vi "Write Startup Views.vi"(9 "View Labels":string[](array[string]), 10 "Startup Views":refnum<class "IViewable.lvclass">[](array[class]), 11 "IViewManager in":refnum<class "IViewManager.lvclass">) -> (3 "IViewManager out":refnum<class "IViewManager.lvclass">)   [LabVIEW 2020, in "IViewManager.lvlib" / "IViewManager.lvclass"]
doc: "写入启动视图"
uses:
  IViewManager.lvclass
  IViewable/IViewable/IViewable.lvclass
  IViewManager Messages/Launch Nested Views Msg/Launch Nested Views Msg.lvclass/Launch Nested Views Msg.ctl
  IViewManager.lvclass/IViewManager.ctl
  IViewManager Messages/Launch Nested Views Msg/Launch Nested Views Msg.lvclass
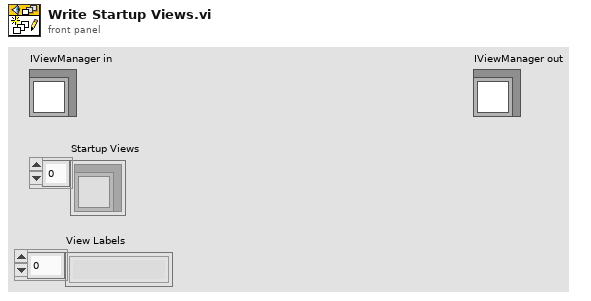
[diagram p1: front panel]
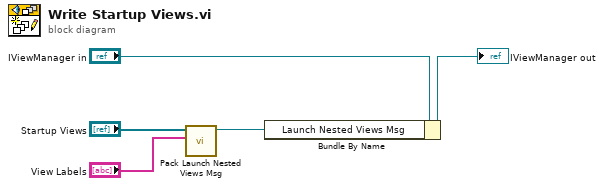
[diagram p0: block diagram]
diagram:
  n1 = call "Pack Launch Nested Views Msg.vi"("View Labels"="View Labels", "Nested Views"="Startup Views") -> ("Launch Nested Views Msg"=w1:refnum<class "Launch Nested Views Msg.lvclass">)  [unwired: 9 in]
  n2 = Bundle By Name(cluster="IViewManager in", "Launch Nested Views Msg"=w1) -> (→"IViewManager out":refnum<class "IViewManager.lvclass">)
